vi "API String - Is Supported Datatype.vi"(9 "error in (no error)":errorcluster, 11 "Data":variant) -> (1 "error out":errorcluster, 2 "Supported Datatype?":bool, 3 "Data(dup)":variant)   [LabVIEW 2017, in "API String Arguments Support.lvlib"]
doc: "Determines whether the data type is a conversion data type supported by API String.\n\n\n> [!NOTE] <b>API String Parameter Support</b>\n>\n> API String parameter support is used to enhance the API parameter functionality of the Communicable State Machine (CSM). API String supports passing various data types in plain text format and is specifically optimized for manual input experiences. API String does not define an argument type. The result obtained via the CSM - Argument Type VI is empty, and it is typically handled in the default case. The following are supported data types:\n> - String\n> - Path\n> - Boolean\n> - Tag\n> - Refnum (including IVI/VISA/UserDefinedRefnumTag)\n> - Integer (I8, I16, I32, I64, U8, U16, U32, U64)\n> - Floating-point (DBL/SGL)\n> - Complex (DBL/SGL)\n> - Timestamp\n> - Enum\n> - Array\n> - Cluster\n> - Other types (represented using CSM-Hexstr)\n>\n> For more details, visit: https://github.com/NEVSTOP-LAB/CSM-API-String-Arguments-Support.\n> You can also refer to the examples. All data types have detailed descriptions and examples.\n\n\n> [!NOTE] <b>CSM HEXSTR Format Argument</b>\n>\n> To pass arbitrary data types in CSM arguments, CSM has a built-in HEXSTR format argument encoding/decoding scheme. The argument type string is HEXSTR. The conversion process is as follows:\n>\n> 1. Convert LabVIEW data to a variant.\n> 2. Serialize the memory image of the variant into a hexadecimal string;\n> 3. Obtain the argument in the form `<HEXSTR> hexadecimal string`, which can be safely embedded in the state string without disrupting CSM message parsing.\n\n\n-- <b>Controls</b> --\n- <b>Data</b>: Input data.\n\n-- <b>Indicators</b> --\n- <b>Data(Dup)</b>: A copy of the input data.\n- <b>Supported Datatype?</b>: Boolean indicating whether API String supports the input data."
uses:
  API String Arguments Support.lvlib
  <vilib>/Utility/Data Type/NI_Data Type.lvlib
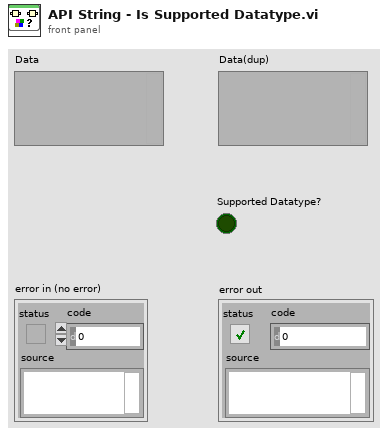
[diagram p1: front panel]
types:
  T1 = typedef "NI_Data Type.lvlib/Data Type.ctl" = enum8{"Invalid Type", "Void", "I8", "I16", "I32", "I64", "U8", "U16", "U32", "U64", "Single Float", "Double Float", "Extended Float", "Single Complex", "Double Complex", "Extended Complex", "Enum U8", "Enum U16", "Enum U32", "Enum U64", "Single Float With Unit", "Double Float With Unit", "Extended Float With Unit", "Single Complex with Unit", "Double Complex with Unit", "Extended Complex with Unit", "Boolean", "String", "Path", "Picture", "Tag", "Array", "Cluster", "Variant", "LV Variant", "Waveform", "Timestamp", "Digital Waveform", "Digital Data", "ExpressData", "Refnum", "External Data", "VI", "Poly VI", "LabVIEW Class Instance", "Fixed Point"}
  T2 = typedef "NI_Data Type.lvlib/Refnum Type.ctl" = enum16{"NotARefnum", "UnknownRefnum", "Generic", "Datalog", "ByteStream", "Device", "Occurence", "TCPNetConnection", "Auto", "Menu", "Imaq", "Hardware", "DataSocket", "Visa", "IVI", "UDPNetConnection", "Notifier", "Queue", "Irda", "EventReg", "DotNet", "UserEvent", "Callback", "UNUSED_EMPTY_POSITION", "BlueToothNetConnection", "LVObjApp", "LVObjVI", "LVObjUnknown", "GenericClass", "UserDefinedRefnumTag", "DataValue", "RT FIFO", "TDMS File"}
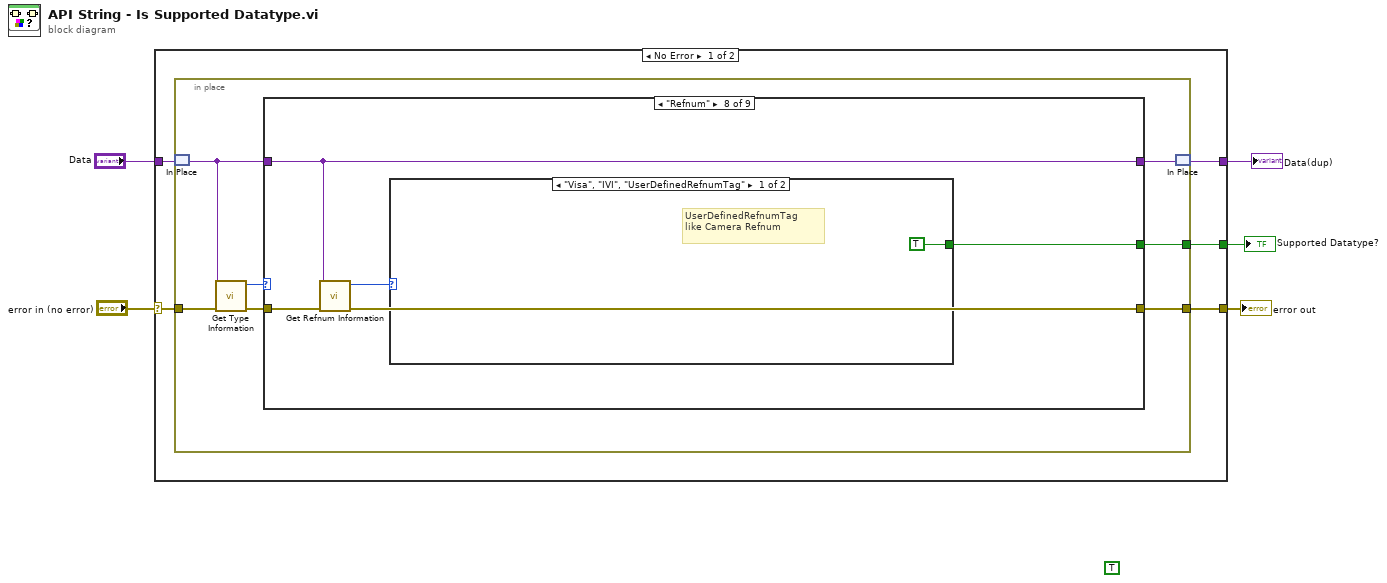
[diagram p0: block diagram]
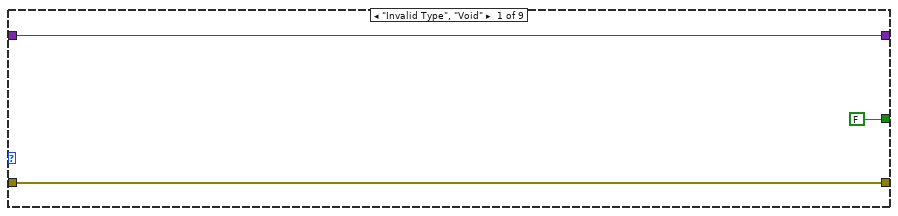
[diagram p2: hidden frame]
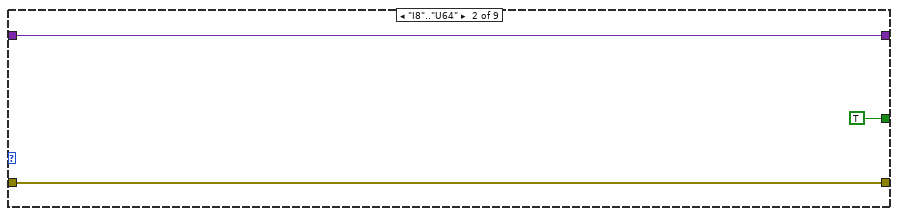
[diagram p3: hidden frame]
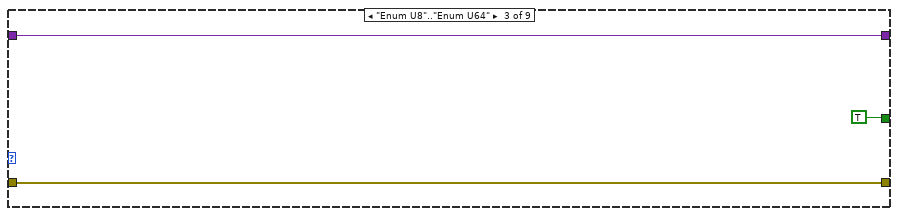
[diagram p4: hidden frame]
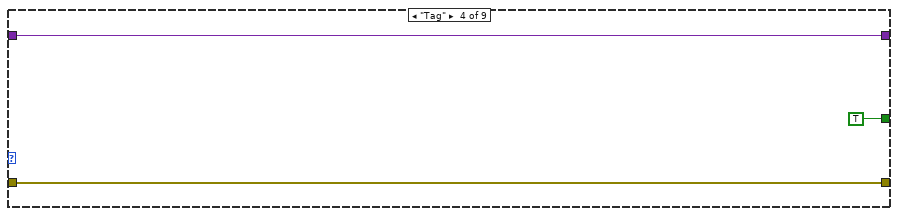
[diagram p5: hidden frame]
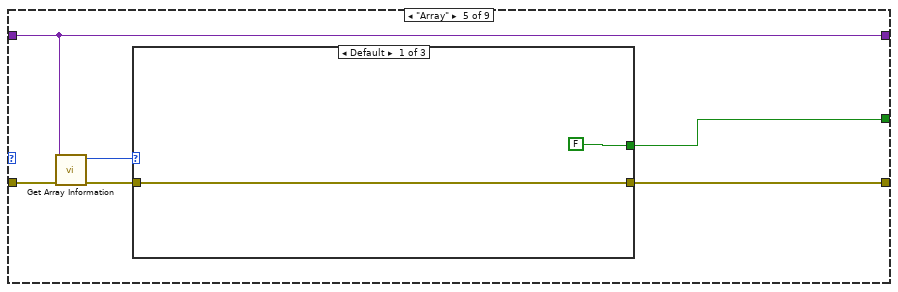
[diagram p6: hidden frame]
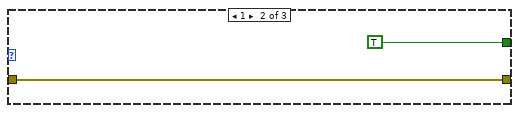
[diagram p7: hidden frame]
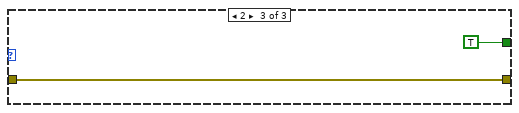
[diagram p8: hidden frame]
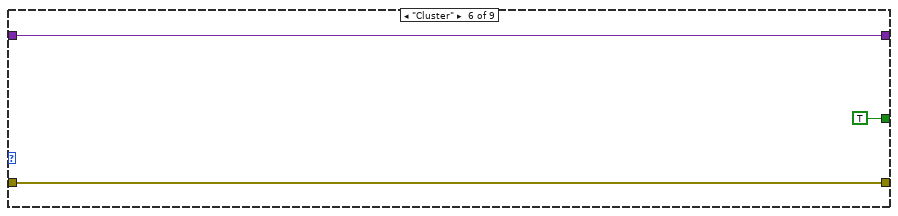
[diagram p9: hidden frame]
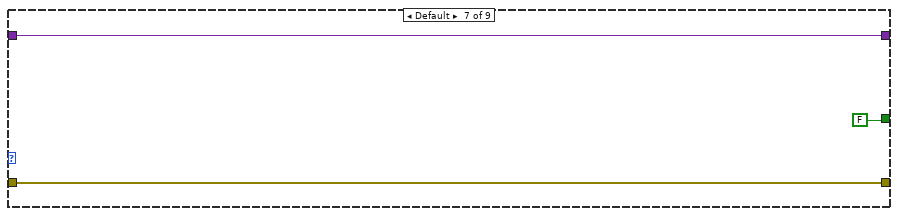
[diagram p10: hidden frame]
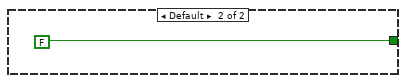
[diagram p11: hidden frame]
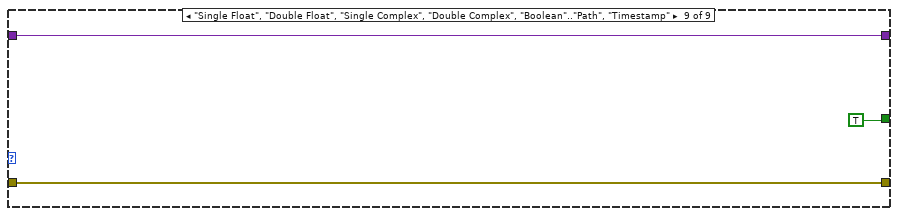
[diagram p12: hidden frame]
diagram:
  (unwired) TRUE
  n1 = case shown="No Error" "error in (no error)" {
    selector: "error in (no error)" -> [w8 w59]
    tunnel: [w10 _] -> w2
    tunnel: "Data" -> [w7 w58]
    tunnel: [w9 w59] -> w4
    tunnel: [w6 w58] -> w1
    frame No Error {
      n2 = in-place {
        in-place-border: [w16] -> w10
        in-place-border: [w14] -> w9
        in-place-border: w8 -> [w13]
        n3 = in-place-match #1(w7) -> (w12:variant)
        n4 = call <vilib>:"Get Type Information.vi"("error in (no error)"=w13, "Variant"=w12) -> ("error out"=w15:errorcluster, "Type"=w17:T1)  [unwired: 5 in, 3 out]
        n5 = case shown="\"Refnum\"" w17 {
          tunnel: [FALSE TRUE TRUE TRUE w31 TRUE FALSE w51 TRUE] -> w16
          tunnel: w12 -> [w19 w21 w25 w27 w30 w43 w45 w48 w56]
          tunnel: w15 -> [w20 w23 w26 w29 w35 w44 w47 w52 w57]
          tunnel: [w20 w23 w26 w29 w33 w44 w47 w50 w57] -> w14
          tunnel: [w19 w21 w25 w27 w30 w43 w45 w48 w56] -> w11
          frame "Invalid Type", "Void" {
          }
          frame "I8".."U64" {
          }
          frame "Enum U8".."Enum U64" {
          }
          frame "Tag" {
          }
          frame "Array" {
            n6 = call <vilib>:"Get Array Information.vi"("error in (no error)"=w35, "Variant"=w30) -> ("error out"=w32:errorcluster, "Number of Dimensions"=w34:i32)  [unwired: 6 in, 2 out]
            n7 = case shown="Default" w34 {
              tunnel: [w36 w38 w40] -> w33
              tunnel: [FALSE TRUE TRUE] -> w31
              tunnel: w32 -> [w36 w38 w40]
              frame Default {
              }
              frame 1 {
              }
              frame 2 {
              }
            }
          }
          frame "Cluster" {
          }
          frame Default {
          }
          frame "Refnum" {
            n8 = call <vilib>:"Get Refnum Information.vi"("error in (no error)"=w52, "Variant"=w48) -> ("error out"=w50:errorcluster, "Reference Type"=w49:T2)  [unwired: 6 in, 2 out]
            n9 = case shown="\"Visa\", \"IVI\", \"UserDefinedRefnumTag\"" w49 {
              tunnel: [TRUE FALSE] -> w51
              frame "Visa", "IVI", "UserDefinedRefnumTag" {
                # "UserDefinedRefnumTag\nlike Camera Refnum"
              }
              frame Default {
              }
            }
          }
          frame "Single Float", "Double Float", "Single Complex", "Double Complex", "Boolean".."Path", "Timestamp" {
          }
        }
        n10 = in-place-match #1(w11) -> (w6:variant)
      }
    }
    frame Error {
    }
  }
  "Data(dup)" <- w1
  "error out" <- w4
  "Supported Datatype?" <- w2
